vi "Extand Listbox.vi"(8 "error in (no error)":errorcluster, 11 "[V] Login in":refnum<class "[V] Login.lvclass">) -> (0 "error out":errorcluster, 3 "[V] Login out":refnum<class "[V] Login.lvclass">)   [LabVIEW 2020, in "[V] Login.lvlib" / "[V] Login.lvclass"]
uses:
  [V] Login.lvclass
  [V] Login.lvclass/[V] Login.ctl
  <vilib>/Analysis/1siggen.llb/Ramp Pattern by Samples.vi
  <vilib>/Analysis/NI_AALBase.lvlib
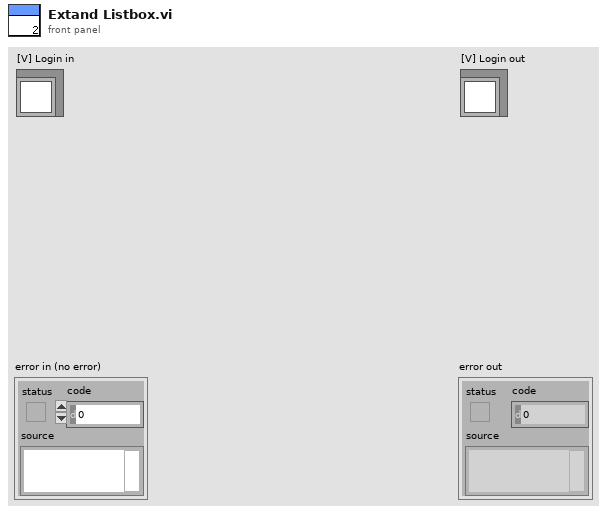
[diagram p1: front panel]
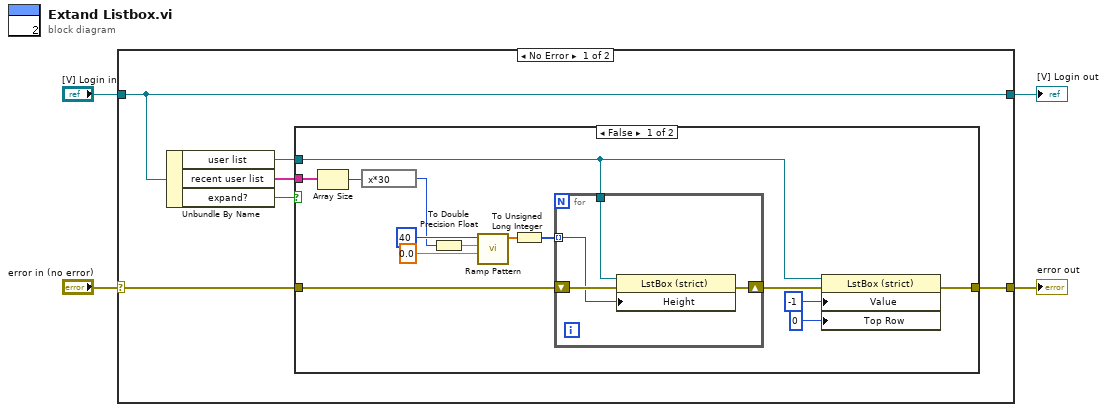
[diagram p0: block diagram]
diagram:
  n1 = case shown="No Error" "error in (no error)" {
    selector: "error in (no error)" -> [w10 w31]
    tunnel: [w8 w31] -> w3
    tunnel: [w9 w30] -> w1
    tunnel: "[V] Login in" -> [w9 w30]
    frame No Error {
      n2 = Unbundle By Name(w9) -> ("user list"=w7:refnum<vi>, "recent user list"=w6:string[], "expand?"=w5:bool)
      n3 = case shown="False" w5 {
        tunnel: w10 -> [w22 w29]
        tunnel: [w18 w29] -> w8
        tunnel: w7 -> [w17 _]
        tunnel: w6 -> [w14 _]
        frame False {
          n4 = Array Size(array=w14) -> (size(s)=w13:i32)
          n5 = expression code="x*30"(w13) -> (w12:i32)
          n6 = To Double Precision Float(number=w12) -> (double precision float=w11:dbl)
          n7 = call-poly <vilib>:"Ramp Pattern.vi"("start"=0.0, "end"=w11, "samples"=40) -> ("Ramp Pattern"=w21:dbl[])  [unwired: 7 in, 1 out]
          n8 = To Unsigned Long Integer(number=w21) -> (unsigned 32bit integer=w20:u32[])
          n9 = for {
            tunnel: w17 -> [w25]
            shift-right: [w27] -> w19
            shift-left: w22 -> [w28]
            tunnel: w20 -> [w26] mode=indexing
            n10 = property class="LstBox (strict)"(reference=w25, error in=w28, "Height"=w26) -> (error out=w27:errorcluster)  [unwired: 1 out]
          }
          n11 = property class="LstBox (strict)"(reference=w17, error in=w19, "Value"=-1, "Top Row"=0) -> (error out=w18:errorcluster)  [unwired: 1 out]
        }
        frame True {
        }
      }
    }
    frame Error {
    }
  }
  "error out" <- w3
  "[V] Login out" <- w1
